vi "DistributePixels.vi"(8 "error in (no error)":errorcluster, 9 "Parameters":T2={"number of planes"=4, "z step"=1.9999999999999998e-05, "pixel dwell time"=1.0000000000000001e-11, "z frequency"=10.0, "number of pixels"=100, "smooth points"=10, "smooth line"=10, "Sine\nSawtooth"=FALSE, "PointSorting"=0, "Sort Points"=FALSE, "X-pixels"=256.0, "Y-lines"=256.0, "pixelstoµm"=256.0, "zoom"=1.0, "Time offset"=1.0000000000000001e-11} {"zoom" min=0.5 step=0.1; "Y-lines" min=1 step=1; "X-pixels" min=1 step=1; "PointSorting" items=["No Difference", "Every Second Point", "Down / Up"]; "smooth line" min=1; "smooth points" min=1; "number of pixels" min=1; "z frequency" format="%_4g"; "number of planes" min=1}, 10 "DutyCluster":T1 {"Iteration" items=["first iteration", "second iteration"]}) -> (0 "error out":errorcluster, 2 "DutyCluster":T1 {"Iteration" items=["first iteration", "second iteration"]}, 3 "x pixels, y pixels, z, time":dbl[][](array[numeric]))   [LabVIEW 2010]
uses:
  <vilib>/Analysis/NI_AALPro.lvlib
  <vilib>/Analysis/_algsub.llb/Real Vector Norm.vi
  TypeDefs/DutyCluster.ctl
  TypeDefs/ParameterCluster.ctl
panel:
  out "break":i32
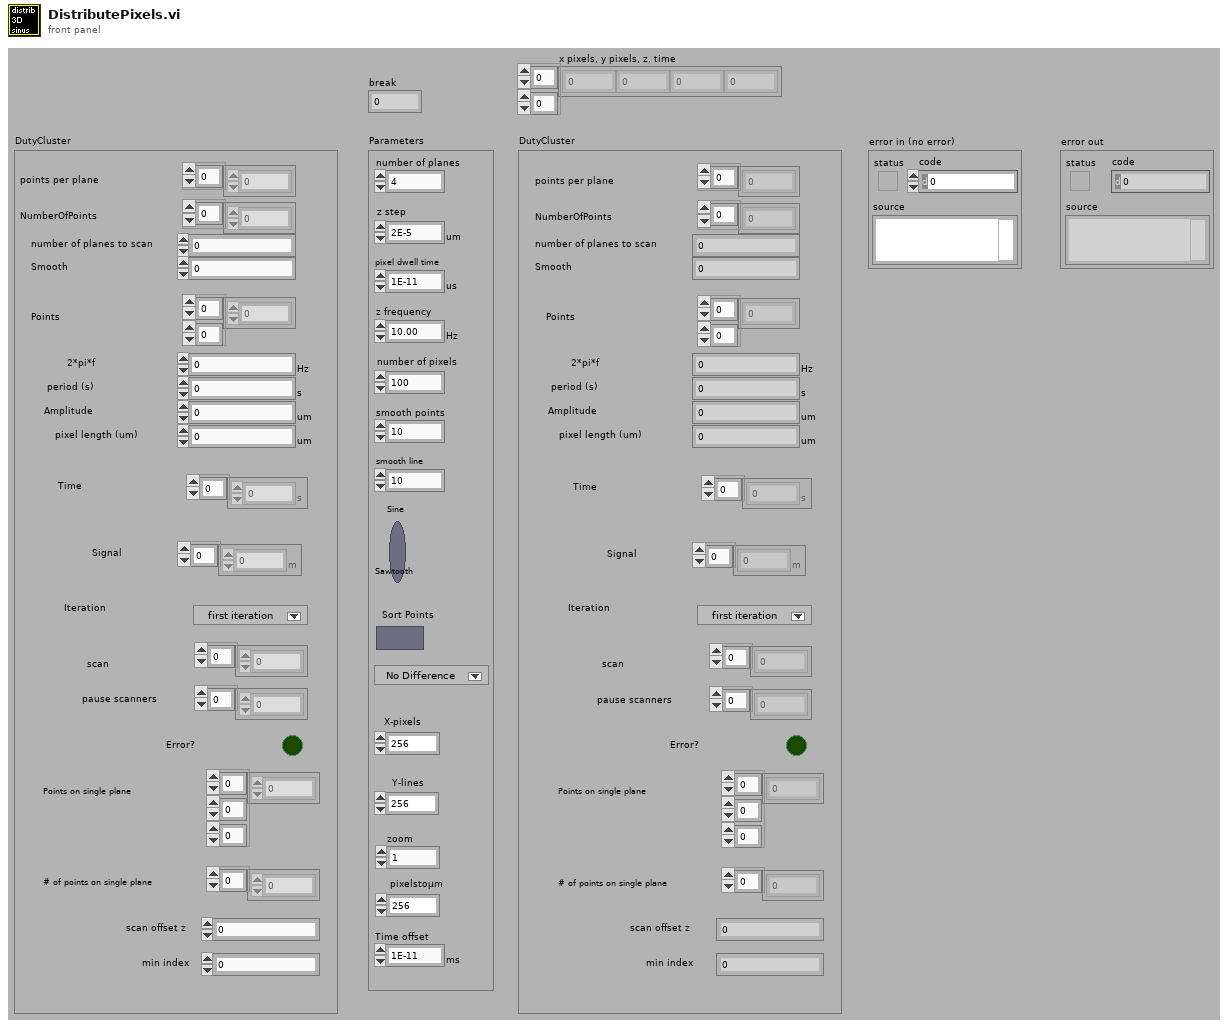
[diagram p1: front panel]
types:
  T1 = typedef "DutyCluster.ctl" = cluster{"points per plane":i32[], "NumberOfPoints":i32[], "number of planes to scan":i32, "Smooth":i32, "Points":dbl[][], "2*pi*f":dbl[unit], "period (s)":dbl[unit], "Amplitude":dbl[unit], "pixel length (um)":dbl[unit], "Time":dbl[unit][], "Signal":dbl[unit][], "Iteration":u16, "scan":i32[], "pause scanners":i32[], "Error?":bool, "Points on single plane":dbl[][][], "# of points on single plane":i32[], "scan offset z":i32, "min index":i32}
  T2 = typedef "ParameterCluster.ctl" = cluster{"number of planes":i32, "z step":dbl[unit], "pixel dwell time":dbl[unit], "z frequency":dbl[unit], "number of pixels":i32, "smooth points":i32, "smooth line":i32, "Sine\nSawtooth":bool, "PointSorting":u16, "Sort Points":bool, "X-pixels":sgl, "Y-lines":sgl, "pixelstoµm":dbl, "zoom":dbl, "Time offset":dbl[unit]}
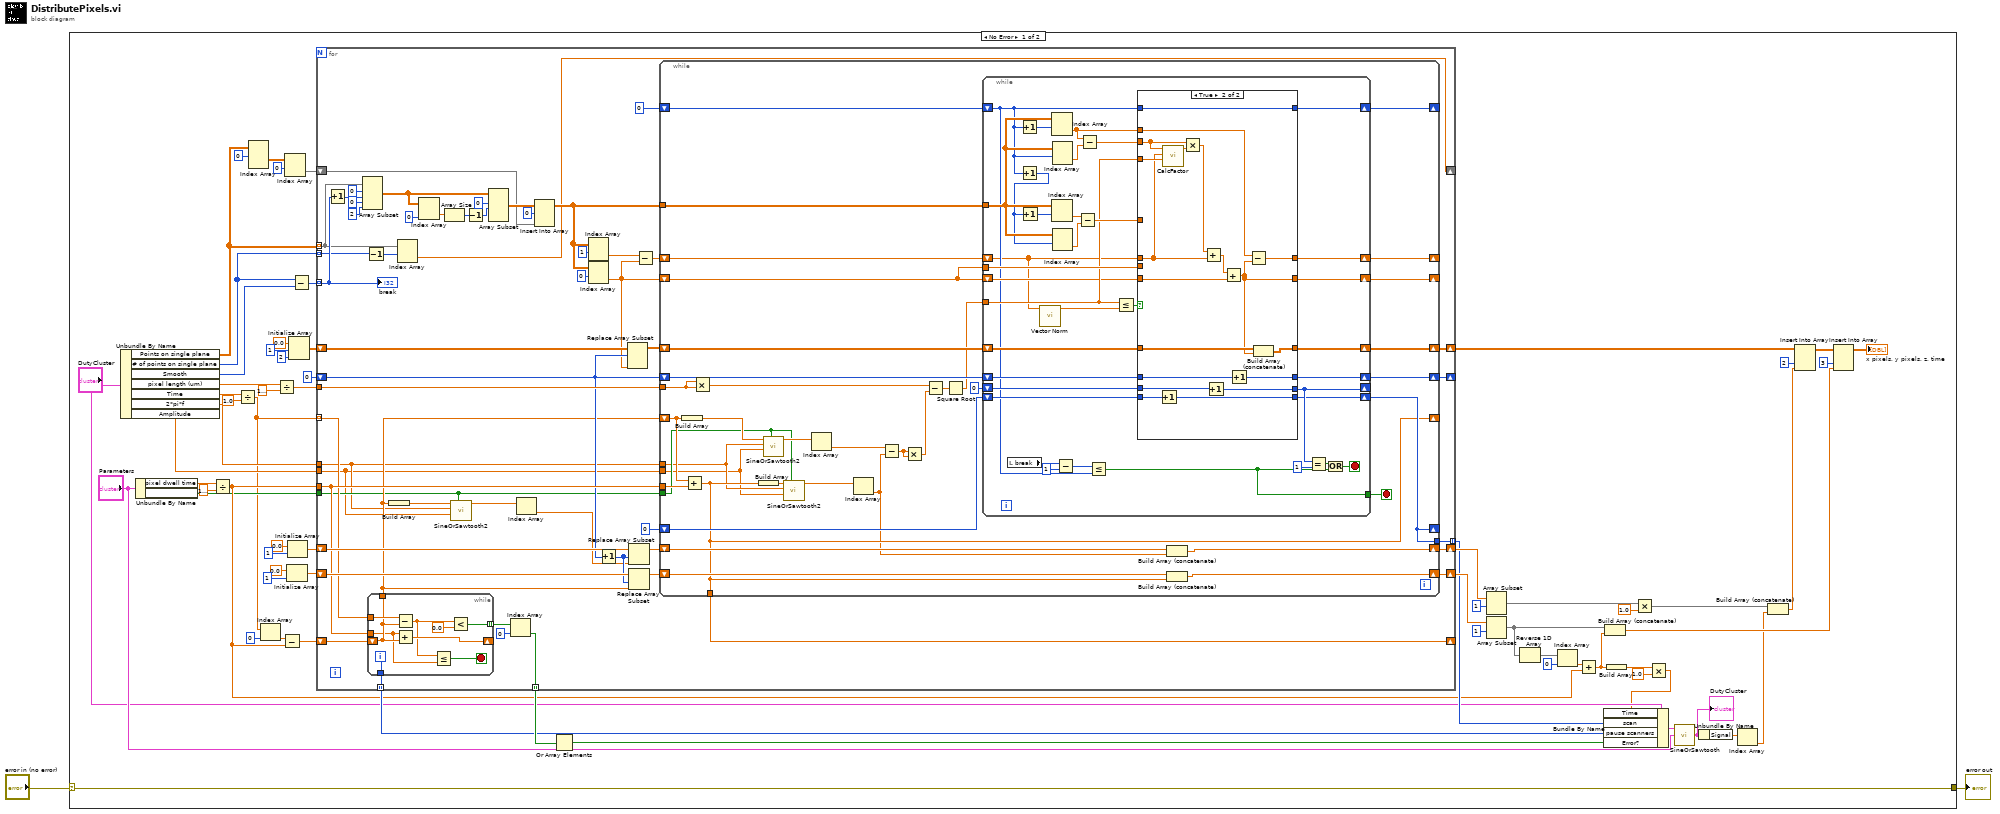
[diagram p0: block diagram]
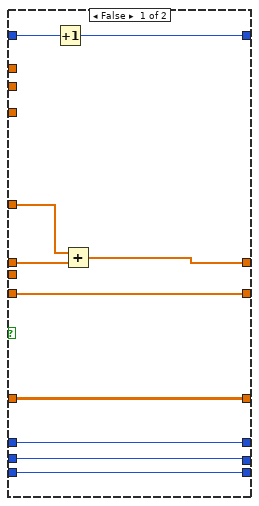
[diagram p2: hidden frame]
diagram:
  n1 = case shown="No Error" "error in (no error)" {
    selector: "error in (no error)" -> [w26 w235]
    tunnel: [w26 w235] -> w1
    frame No Error {
      n2 = Unbundle By Name("DutyCluster") -> ("Points on single plane"=w24:dbl[][][], "# of points on single plane"=w25:i32[], "Smooth"=w36:i32, "pixel length (um)"=w22:dbl[unit], "Time"=w10:dbl[unit][], "2*pi*f"=w16:dbl[unit], "Amplitude"=w15:dbl[unit])
      n3 = Unbundle By Name("Parameters") -> ("pixel dwell time"=w18:dbl[unit], "Sine\nSawtooth"=w14:bool)
      n4 = Divide(x=w18, y=dbl[unit] 1e-06) -> (x/y=w17:dbl)
      n5 = Divide(x=w10, y=dbl[unit] 1.0) -> (x/y=w9:dbl[])
      n6 = Index Array(array=w24, index (dim 0)=0 ("index (page)")) -> (element=w51:dbl[][])  [unwired: 2 in]
      n7 = Index Array(array=w9, index=0) -> (element=w49:dbl)
      n8 = Divide(x=w22, y=dbl[unit] 1e-06) -> (x/y=w21:dbl)
      n9 = Subtract(x=w49, y=w17) -> (x-y=w35:dbl)
      n10 = Index Array(array=w51, index (row)=0) -> (element=w50:dbl[])  [unwired: 1 in]
      n11 = Initialize Array(0.0 ("element"), 1 ("dimension size")) -> (w34:dbl[])
      n12 = Initialize Array(0.0 ("element"), 1 ("dimension size")) -> (w33:dbl[])
      n13 = Initialize Array(0.0 ("element"), 1 ("dimension size"), 2 ("dimension size")) -> (w65:dbl[][])
      n14 = Subtract(x=w25, y=w36) -> (x-y=w54:i32[])
      n15 = for {
        shift-right: [w108] -> w62
        shift-left: w65 -> [w106]
        tunnel: w24 -> [w90] mode=indexing
        tunnel: w9 -> [w76] mode=indexing
        tunnel: w17 -> [w84]
        tunnel: w21 -> [w122]
        shift-right: [w121] -> _
        shift-left: 0 -> [w83]
        tunnel: w54 -> [w92] mode=indexing
        shift-right: [w103] -> w46
        shift-left: w33 -> [w105]
        shift-right: [w100] -> w45
        shift-left: w34 -> [w101]
        shift-right: [w85] -> _
        shift-left: w35 -> [w95]
        tunnel: [w94] -> w27 mode=indexing
        tunnel: [w93] -> w28 mode=indexing
        tunnel: w25 -> [w89] mode=indexing
        shift-right: [w87] -> _
        shift-left: w50 -> [w86]
        tunnel: [w80] -> w38 mode=indexing
        tunnel: w16 -> [w71]
        tunnel: w15 -> [w70]
        tunnel: w14 -> [w72]
        n16 = Increment(x=w92) -> (x+1=w91:i32)
        n17 = Array Subset(array=w90, index (row)=0 ("index"), length (row)=w91, index (col)=0 ("index"), length (col)=2 ("length")) -> (w114:dbl[][])
        n18 = Decrement(x=w89) -> (x-1=w88:i32)
        n19 = while {
          shift-right: [w129] -> _
          shift-left: w95 -> [w131]
          tunnel: w84 -> [w128]
          tunnel: w76 -> [w132]
          tunnel: [w133] -> w94
          tunnel: [w131] -> w78
          tunnel: [w125] -> w79 mode=indexing
          i -> [w133]
          stop <- w130 stop-if-true
          n20 = Subtract(x=w132, y=w131) -> (x-y=w127:dbl)
          n21 = Add(x=w128, y=w131) -> (x+y=w129:dbl)
          n22 = Less Or Equal?(x=w127, y=w128) -> (x <= y?=w130:bool)
          n23 = Less?(x=w127, y=0.0) -> (x < y?=w125:bool)
        }
        n24 = Build Array(w78) -> (w74:dbl[])
        n25 = Index Array(array=w90, index (row)=w88) -> (element=w87:dbl[])  [unwired: 1 in]
        n26 = Index Array(array=w114, index (col)=0 ("disabled index (col)")) -> (element=w117:dbl[])  [unwired: 1 in]
        n27 = Array Size(array=w117) -> (size(s)=w115:i32)
        n28 = call "SineOrSawtooth2.vi"("Sine\nSawtooth"=w72, "Amplitude"=w70, "2*pi*f"=w71, "Time"=w74) -> ("Signal"=w73:dbl[])  [unwired: 6 in, 1 out]
        n29 = Decrement(x=w115) -> (x-1=w113:i32)
        n30 = Array Subset(array=w114, index (row)=0 ("index"), length (row)=w113) -> (w97:dbl[][])  [unwired: 2 in]
        n31 = Index Array(array=w79, index=0) -> (element=w80:bool)
        n32 = Index Array(array=w73) -> (element=w75:dbl)  [unwired: 1 in]
        n33 = Insert Into Array(array=w97, index (row)=0, new element=w86) -> (w96:dbl[][])  [unwired: 1 in]
        n34 = Index Array(array=w96, index (row)=1) -> (element=w110:dbl[])  [unwired: 1 in]
        n35 = Index Array(array=w96, index (row)=0) -> (element=w77:dbl[])  [unwired: 1 in]
        n36 = Increment(x=w83) -> (x+1=w82:i32)
        n37 = Replace Array Subset(array=w106, new element=w77, index (row)=w83) -> (w107:dbl[][])  [unwired: 1 in]
        n38 = Replace Array Subset(array=w105, new element=w75, index=w82) -> (w104:dbl[])
        n39 = Replace Array Subset(array=w101, new element=w78, index=w82) -> (w102:dbl[])
        n40 = Subtract(x=w110, y=w77) -> (x-y=w109:dbl[])
        n41 = while {
          tunnel: w96 -> [w163]
          shift-right: [w144] -> _
          shift-left: w78 -> [w145]
          tunnel: w84 -> [w170]
          tunnel: w122 -> [w154]
          shift-right: [w161] -> w121
          shift-left: w83 -> [w165]
          shift-right: [w143] -> w108
          shift-left: w107 -> [w162]
          shift-right: [w158] -> _
          shift-left: 0 -> [w159]
          shift-right: [w157] -> _
          shift-left: w77 -> [w160]
          shift-right: [w155] -> _
          shift-left: w109 -> [w156]
          shift-right: [w150] -> w103
          shift-left: w104 -> [w151]
          shift-right: [w148] -> w100
          shift-left: w102 -> [w149]
          shift-right: [w146] -> _
          shift-left: 0 ("index (row)") -> [w147]
          tunnel: [w144] -> w85
          tunnel: [w146] -> w93
          tunnel: w72 -> [w136]
          tunnel: w71 -> [w135]
          tunnel: w70 -> [w134]
          stop <- w152 stop-if-true
          n42 = Build Array(w145) -> (w140:dbl[])
          n43 = Add(x=w145, y=w170) -> (x+y=w144:dbl)
          n44 = Multiply(x=w154, y=w154) -> (x*y=w168:dbl)
          n45 = Build Array(w144) -> (w139:dbl[])
          n46 = call "SineOrSawtooth2.vi"("Sine\nSawtooth"=w136, "Amplitude"=w134, "2*pi*f"=w135, "Time"=w140) -> ("Signal"=w138:dbl[])  [unwired: 6 in, 1 out]
          n47 = call "SineOrSawtooth2.vi"("Sine\nSawtooth"=w136, "Amplitude"=w134, "2*pi*f"=w135, "Time"=w139) -> ("Signal"=w137:dbl[])  [unwired: 6 in, 1 out]
          n48 = Index Array(array=w138) -> (element=w141:dbl)  [unwired: 1 in]
          n49 = Index Array(array=w137) -> (element=w142:dbl)  [unwired: 1 in]
          n50 = Subtract(x=w141, y=w142) -> (x-y=w169:dbl)
          n51 = Multiply(x=w169, y=w169) -> (x*y=w167:dbl)
          n52 = Subtract(x=w168, y=w167) -> (x-y=w166:dbl)
          n53 = Square Root(x=w166) -> (sqrt(x)=w153:dbl)
          n54 = while {
            tunnel: w163 -> [w186]
            tunnel: w153 -> [w187]
            shift-right: [w204] -> w157
            shift-left: w160 -> [w185]
            shift-right: [w205] -> w155
            shift-left: w156 -> [w172]
            shift-right: [w188] -> w143
            shift-left: w162 -> [w203]
            shift-right: [w202] -> w158
            shift-left: w159 -> [w180]
            tunnel: w160 -> [w193]
            shift-right: [w190] -> _
            shift-left: 0 -> [w191]
            shift-right: [w189] -> w161
            shift-left: w165 -> [w183]
            tunnel: [w176] -> w152
            shift-right: [w182] -> w146
            shift-left: w147 -> [w181]
            stop <- w174 stop-if-true
            n55 = local read "break"() -> (w177:i32)
            n56 = Increment(x=w180) -> (x+1=w200:i32)
            n57 = Increment(x=w180) -> (x+1=w184:i32)
            n58 = Increment(x=w184) -> (x+1=w197:i32)
            n59 = call-poly <vilib>:"Vector Norm.vi"("Input Vector"=w172) -> ("norm"=w171:dbl)  [unwired: 9 in, 1 out]
            n60 = Index Array(array=w186, index (row)=w200) -> (element=w194:dbl[])  [unwired: 1 in]
            n61 = Index Array(array=w186, index (row)=w197) -> (element=w196:dbl[])  [unwired: 1 in]
            n62 = Index Array(array=w186, index (row)=w180) -> (element=w201:dbl[])  [unwired: 1 in]
            n63 = Index Array(array=w186, index (row)=w184) -> (element=w198:dbl[])  [unwired: 1 in]
            n64 = Subtract(x=w177, y=1) -> (x-y=w179:i32)
            n65 = Subtract(x=w196, y=w198) -> (x-y=w195:dbl[])
            n66 = Subtract(x=w194, y=w201) -> (x-y=w173:dbl[])
            n67 = Less Or Equal?(x=w179, y=w180) -> (x <= y?=w176:bool)
            n68 = Less Or Equal?(x=w187, y=w171) -> (x <= y?=w199:bool)
            n69 = case shown="True" w199 {
              tunnel: w172 -> [w210 w216]
              tunnel: w195 -> [w209 _]
              tunnel: [w214 w219] -> w205
              tunnel: w173 -> [_ w218]
              tunnel: w185 -> [w213 w234]
              tunnel: [w213 w223] -> w204
              tunnel: w183 -> [w212 w233]
              tunnel: w203 -> [w211 w224]
              tunnel: [w212 w232] -> w189
              tunnel: [w211 w225] -> w188
              tunnel: w180 -> [w208 w231]
              tunnel: [w215 w231] -> w202
              tunnel: w187 -> [_ w217]
              tunnel: w194 -> [_ w228]
              tunnel: w193 -> [_ _]
              tunnel: w191 -> [w207 w227]
              tunnel: [w207 w226] -> w190
              tunnel: w181 -> [w206 w222]
              tunnel: [w206 w221] -> w182
              frame False {
                n70 = Increment(x=w208) -> (x+1=w215:i32)
                n71 = Add(x=w209, y=w210) -> (x+y=w214:dbl[])
              }
              frame True {
                n72 = Increment(x=w222) -> (x+1=w221:i32)
                n73 = call "CalcFactor.vi"("delta"=w217, "deltavec"=w216, "point"=w218) -> ("factor"=w220:dbl)  [unwired: 5 in, 1 out]
                n74 = Multiply(x=w218, y=w220) -> (x*y=w229:dbl[])
                n75 = Add(x=w229, y=w216) -> (x+y=w230:dbl[])
                n76 = Increment(x=w227) -> (x+1=w226:i32)
                n77 = Add(x=w230, y=w234) -> (x+y=w223:dbl[])
                n78 = Increment(x=w233) -> (x+1=w232:i32)
                n79 = Subtract(x=w228, y=w223) -> (x-y=w219:dbl[])
                n80 = Build Array (concatenate)(w224, w223) -> (w225:dbl[][])
              }
            }
            n81 = Equal?(x=w190, y=1) -> (x = y?=w175:bool)
            n82 = Or(x=w175, y=w176) -> (x .or. y?=w174:bool)
          }
          n83 = Build Array (concatenate)(w151, w142) -> (w150:dbl[])
          n84 = Build Array (concatenate)(w149, w144) -> (w148:dbl[])
        }
        "break" <- w92
      }
      n85 = Or Array Elements(Boolean array=w38) -> (logical OR=w29:bool)
      n86 = Array Subset(array=w46, index=1) -> (w4:dbl[])  [unwired: 1 in]
      n87 = Array Subset(array=w45, index=1) -> (w41:dbl[])  [unwired: 1 in]
      n88 = Reverse 1D Array(array=w41) -> (reversed array=w44:dbl[])
      n89 = Index Array(array=w44, index=0) -> (element=w42:dbl)
      n90 = Add(x=w42, y=w17) -> (x+y=w37:dbl)
      n91 = Build Array (concatenate)(w41, w37) -> (w39:dbl[])
      n92 = Build Array(w37) -> (w7:dbl[])
      n93 = Multiply(x=w4, y=dbl[unit] 1.0) -> (x*y=w3:dbl[unit][])
      n94 = Multiply(x=w7, y=dbl[unit] 1.0) -> (x*y=w6:dbl[unit][])
      n95 = Bundle By Name(cluster="DutyCluster", "Time"=w6, "scan"=w28, "pause scanners"=w27, "Error?"=w29) -> (w31:T1)
      n96 = call "SineOrSawtooth.vi"("Parameters"="Parameters", "DutyCluster"=w31) -> ("DutyCluster"=w12:T1)  [unwired: 2 in, 1 out]
      "DutyCluster" <- w12
      n97 = Unbundle By Name(w12) -> ("Signal"=w32:dbl[unit][])
      n98 = Index Array(array=w32) -> (element=w20:dbl[unit])  [unwired: 1 in]
      n99 = Build Array (concatenate)(w3, w20) -> (w40:dbl[unit][])
      n100 = Insert Into Array(array=w62, index (col)=2 ("disabled index (col)"), new element=w40) -> (w56:dbl[][])  [unwired: 1 in]
      n101 = Insert Into Array(array=w56, index (col)=3 ("disabled index (col)"), new element=w39) -> (→"x pixels, y pixels, z, time":dbl[][])  [unwired: 1 in]
    }
    frame Error {
    }
  }
  "error out" <- w1
